vi "9603 Keyname empty--error.vi"(8 "error in":errorcluster) -> (0 "error out":errorcluster)   [LabVIEW 2019, in "Electronic Datasheet.lvlib"]
uses:
  Electronic Datasheet.lvlib
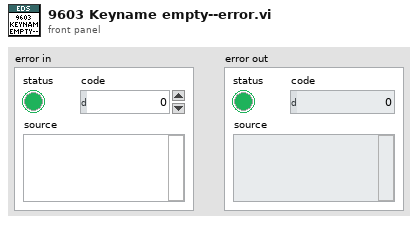
[diagram p1: front panel]
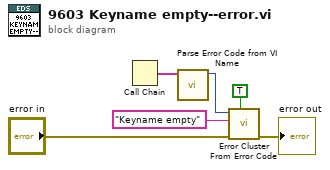
[diagram p0: block diagram]
diagram:
  n1 = Call Chain() -> (call chain=w1:string[])
  n2 = call "Parse Error Code from VI Name.vi"("Call Chain"=w1) -> ("Error Code"=w2:i32)  [unwired: 10 in]
  n3 = call <vilib>:"Error Cluster From Error Code.vi"("show call chain? (False)"=TRUE, "error in (no error)"="error in", "error message (\"\")"="Keyname empty" ("error message (\"\")"), "error code (0)"=w2) -> ("error out"=→"error out":errorcluster)  [unwired: 5 in]
